vi "Project Parser_Identify Internal Dependencies.vi"(7 "To Lower Case?(T)":bool=TRUE, 10 "Internal Relative Paths":string[](array[string]), 11 "Internal Target Map":map{string, string}(c390)) -> (3 "Found Internal Dependencies":string[](array[string]))   [LabVIEW 2019, in "Project.Dependencies Finder.lvlib"]
doc: "Find longest path matches and identify the corresponding dependencies.\n\n2020-11-13: Henrik Dueholm Hansen"
uses:
  de6743d0-67f7-4fc9-ad23-fab93be5b0c6.vi
  Project.Dependencies Finder.lvlib
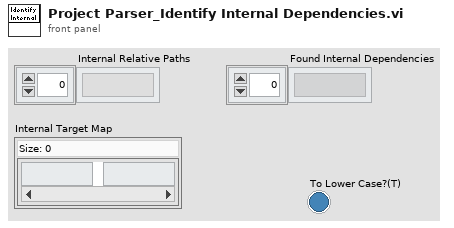
[diagram p1: front panel]
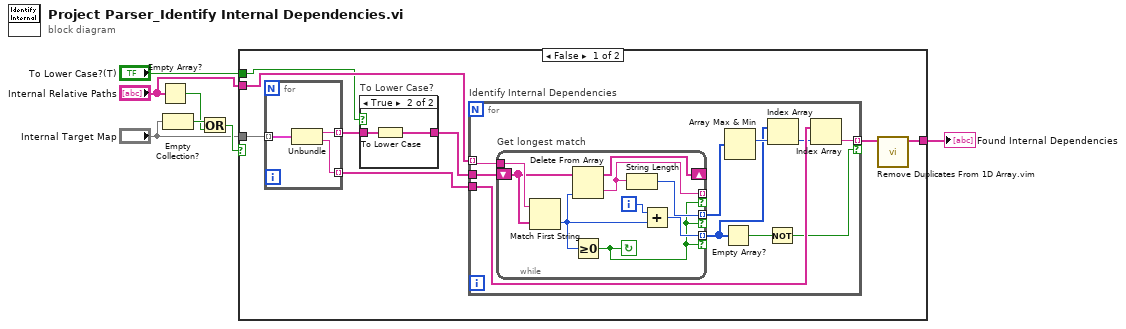
[diagram p0: block diagram]
diagram:
  n1 = Empty Array?(array="Internal Relative Paths") -> (empty?=w4:bool)
  n2 = Empty Collection?(1:"Internal Target Map") -> (0:w6:bool)
  n3 = Or(x=w6, y=w4) -> (x .or. y?=w7:bool)
  n4 = case shown="False" w7 {
    tunnel: "Internal Relative Paths" -> [w14 _]
    tunnel: [w10 _] -> w2
    tunnel: "Internal Target Map" -> [w9 _]
    tunnel: "To Lower Case?(T)" -> [w8 _]
    frame False {
      n5 = for {
        tunnel: w9 -> [w40] mode=indexing
        tunnel: [w39] -> w15 mode=indexing
        tunnel: [w38] -> w12 mode=indexing
        n6 = Unbundle(w40) -> ("Directory Target"=w39:string, "Dependency Name"=w38:string)
      }
      n7 = case "To Lower Case?" shown="True" w8 {
        tunnel: w15 -> [w16 w18]
        tunnel: [w16 w17] -> w13
        frame False {
        }
        frame True {
          n8 = To Lower Case(string=w18) -> (all lower case string=w17:string[])
        }
      }
      n9 = for "Identify Internal Dependencies" {
        tunnel: w14 -> [w28] mode=indexing
        tunnel: [w25] -> w11 mode=indexing if=w19
        tunnel: w13 -> [w27]
        tunnel: w12 -> [w26]
        n10 = while "Get longest match" {
          tunnel: w28 -> [w37]
          shift-right: [w34] -> _
          shift-left: w27 -> [w36]
          tunnel: [w33] -> w21 mode=indexing if=w29
          tunnel: [w31] -> _ mode=indexing if=w29
          tunnel: [w30] -> w24 mode=indexing if=w29
          i -> [w32]
          stop <- w29 continue-if-true
          n11 = Match First String(2:w36, 3:w37) -> (0:w35:i32)  [unwired: 1 out]
          n12 = Delete From Array(array=w36, index=w35) -> (deleted portion=w31:string, array with subset deleted=w34:string[])  [unwired: 1 in]
          n13 = Greater Or Equal To 0?(x=w35) -> (x >= 0?=w29:bool)
          n14 = String Length(string=w31) -> (length=w30:i32)
          n15 = Add(x=w32, y=w35) -> (x+y=w33:i32)
        }
        n16 = Empty Array?(array=w21) -> (empty?=w20:bool)
        n17 = Array Max & Min(array=w24) -> (max index (indices)=w23:i32)  [unwired: 3 out]
        n18 = Not(x=w20) -> (.not. x?=w19:bool)
        n19 = Index Array(array=w21, index=w23) -> (element=w22:i32)
        n20 = Index Array(array=w26, index=w22) -> (element=w25:string)
      }
      n21 = call "Remove Duplicates From 1D Array.vim"("array"=w11) -> ("array with duplicates removed"=w10:string[])  [unwired: 10 in]
    }
    frame True {
    }
  }
  "Found Internal Dependencies" <- w2
